vi "CalculateDistances.vi"(6 "isReverse?":bool, 10 "Landmarkers Coordinates":u32[][](array[numeric])=[[0, 0, 0], [0, 0, 0], [0, 0, 0], [0, 0, 0], [0, 0, 0], [0, 0, 0], [0, 0, 0], [0, 0, 0], [0, 0, 0], [0, 0, 0], [0, 0, 0], [0, 0, 0], [0, 0, 0], [0, 0, 0], [0, 0, 0], [0, 0, 0], [0, 0, 0], [0, 0, 0], [0, 0, 0], [0, 0, 0], [0, 0, 0]], 11 "Antenna Coordinates":u32[][](array[numeric])) -> (3 "Distances":dbl[](array[numeric]))   [LabVIEW 2024]
uses:
  <vilib>/vision/NI_Vision_Development_Module.lvlib
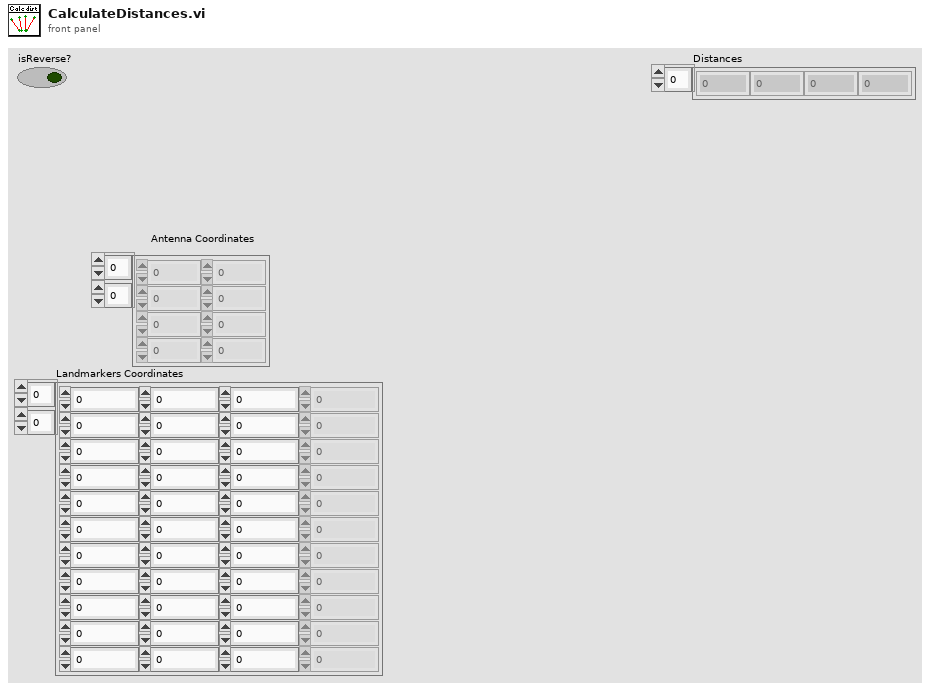
[diagram p1: front panel]
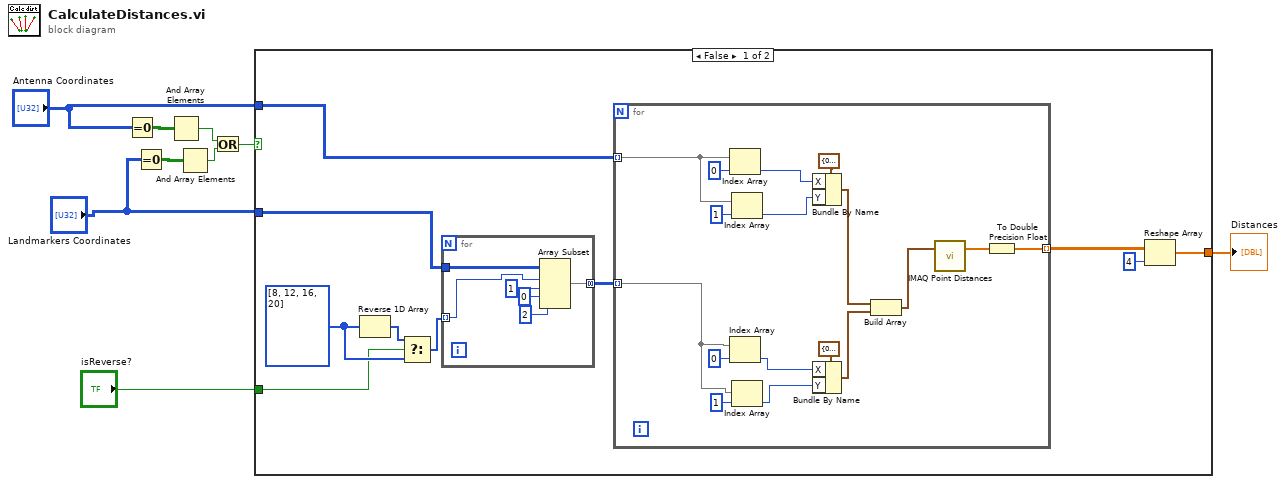
[diagram p0: block diagram]
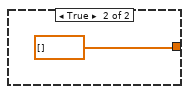
[diagram p2: hidden frame]
diagram:
  n1 = Equal To 0?(x="Antenna Coordinates") -> (x = 0?=w8:bool[][])
  n2 = Equal To 0?(x="Landmarkers Coordinates") -> (x = 0?=w7:bool[][])
  n3 = And Array Elements(Boolean array=w8) -> (logical AND=w5:bool)
  n4 = And Array Elements(Boolean array=w7) -> (logical AND=w4:bool)
  n5 = Or(x=w5, y=w4) -> (x .or. y?=w6:bool)
  n6 = case shown="False" w6 {
    tunnel: "Antenna Coordinates" -> [w19 _]
    tunnel: "Landmarkers Coordinates" -> [w15 _]
    tunnel: "isReverse?" -> [w13 _]
    tunnel: [w11 dbl[] [] ("Distances")] -> w1
    frame False {
      w17 = i32[] [8, 12, 16, 20]
      n7 = Reverse 1D Array(array=w17) -> (reversed array=w16:i32[])
      n8 = Select(t=w16, s=w13, f=w17) -> (s? t:f=w18:i32[])
      n9 = for {
        tunnel: w18 -> [w24] mode=indexing
        tunnel: [w23] -> w14 mode=concatenating
        tunnel: w15 -> [w22]
        n10 = Array Subset(array=w22, index (row)=w24, length (row)=1 ("length"), index (col)=0 ("index"), length (col)=2 ("length")) -> (w23:u32[][])
      }
      n11 = for {
        tunnel: w19 -> [w39] mode=indexing
        tunnel: w14 -> [w33] mode=indexing
        tunnel: [w26] -> w12 mode=indexing
        n12 = Index Array(array=w39, index=0) -> (element=w38:u32)
        n13 = Index Array(array=w33, index=0) -> (element=w32:u32)
        n14 = Index Array(array=w39, index=1) -> (element=w37:u32)
        n15 = Index Array(array=w33, index=1) -> (element=w31:u32)
        n16 = Bundle By Name(cluster=cluster{"X":sgl, "Y":sgl} {"X"=0.0, "Y"=0.0}, "X"=w38, "Y"=w37) -> (w30:cluster{"X":sgl, "Y":sgl})
        n17 = Bundle By Name(cluster=cluster{"X":sgl, "Y":sgl} {"X"=0.0, "Y"=0.0}, "X"=w32, "Y"=w31) -> (w29:cluster{"X":sgl, "Y":sgl})
        n18 = Build Array(w30, w29) -> (w28:cluster{"X":sgl, "Y":sgl}[])
        n19 = call "IMAQ Point Distances"("Points"=w28) -> ("Distances"=w27:sgl[])  [unwired: 4 in, 1 out]
        n20 = To Double Precision Float(number=w27) -> (double precision float=w26:dbl[])
      }
      n21 = Reshape Array(w12, 4 ("dimension size")) -> (w11:dbl[])
    }
    frame True {
    }
  }
  "Distances" <- w1
